vi "SW-Modbus Err Status.vi"(11 "Modbus Error Code function":i32) -> (2 "结果输出":string, 3 "Status":bool)   [LabVIEW 2015]
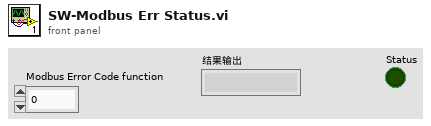
[diagram p1: front panel]
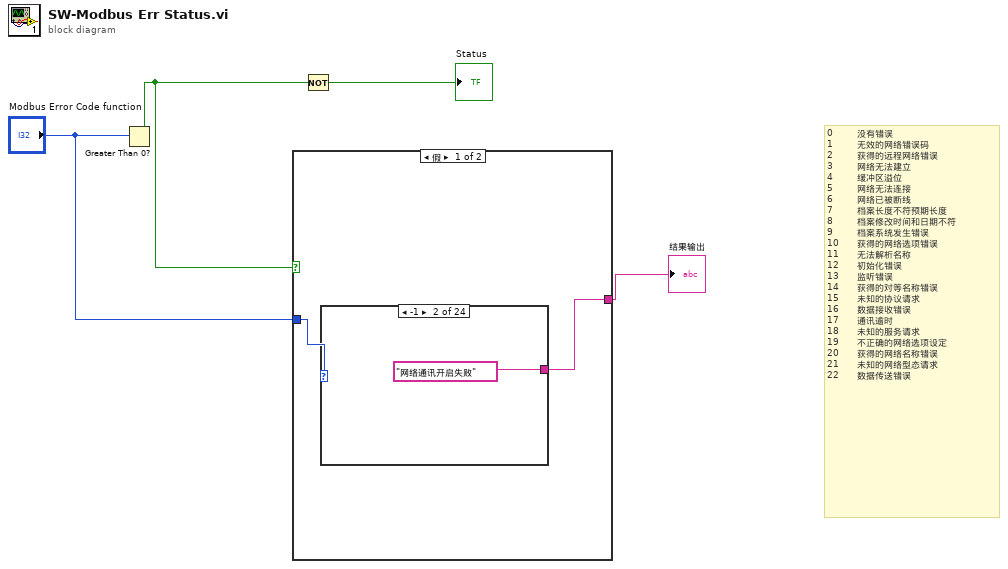
[diagram p0: block diagram]
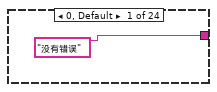
[diagram p2: hidden frame]
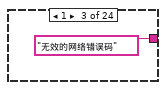
[diagram p3: hidden frame]
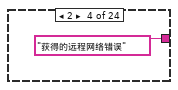
[diagram p4: hidden frame]
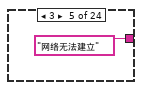
[diagram p5: hidden frame]
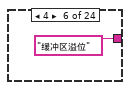
[diagram p6: hidden frame]
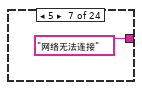
[diagram p7: hidden frame]
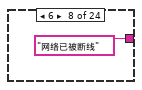
[diagram p8: hidden frame]
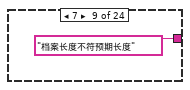
[diagram p9: hidden frame]
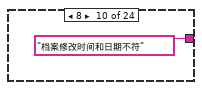
[diagram p10: hidden frame]
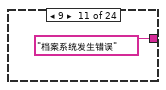
[diagram p11: hidden frame]
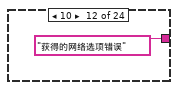
[diagram p12: hidden frame]
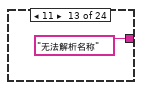
[diagram p13: hidden frame]
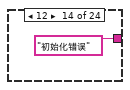
[diagram p14: hidden frame]
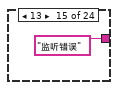
[diagram p15: hidden frame]
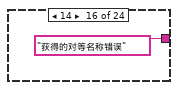
[diagram p16: hidden frame]
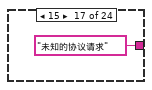
[diagram p17: hidden frame]
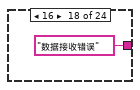
[diagram p18: hidden frame]
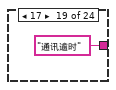
[diagram p19: hidden frame]
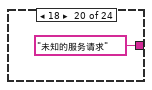
[diagram p20: hidden frame]
diagram:
  # "0        没有错误\n1        无效的网络错误码\n2        获得的远程网络错误\n3        网络无法建立\n4        缓冲区溢位\n5        网络无法连接\n6        网络已被断线\n7        档案长度不符预期长度\n8        档案修改时间和日期不符\n9        档案系统发生错误\n10      获得的网络选项错误\n11      无法解析名称\n12      初始化错误\n13      监听错误\n14      获得的对等名称错误\n15      未知的协议请求\n16      数据接收错误\n17      通讯逾时\n18      未知的服务请求\n19      不正确的网络选项设定\n20      获得的网络名称错误\n21      未知的网络型态请求\n22      数据传送错误"
  n1 = Greater Than 0?(x="Modbus Error Code function") -> (x > 0?=w2:bool)
  n2 = case shown="假" w2 {
    tunnel: "Modbus Error Code function" -> [w6 _]
    tunnel: [w5 "没有错误"] -> w3
    frame False {
      n3 = case shown="-1" w6 {
        tunnel: ["没有错误" "网络通讯开启失败" "无效的网络错误码" "获得的远程网络错误" "网络无法建立" "缓冲区溢位" "网络无法连接" "网络已被断线" "档案长度不符预期长度" "档案修改时间和日期不符" "档案系统发生错误" "获得的网络选项错误" "无法解析名称" "初始化错误" "监听错误" "获得的对等名称错误" "未知的协议请求" "数据接收错误" "通讯逾时" "未知的服务请求" "不正确的网络选项设定" "获得的网络名称错误" "未知的网络型态请求" "数据传送错误"] -> w5
        frame 0, Default {
        }
        frame -1 {
        }
        frame 1 {
        }
        frame 2 {
        }
        frame 3 {
        }
        frame 4 {
        }
        frame 5 {
        }
        frame 6 {
        }
        frame 7 {
        }
        frame 8 {
        }
        frame 9 {
        }
        frame 10 {
        }
        frame 11 {
        }
        frame 12 {
        }
        frame 13 {
        }
        frame 14 {
        }
        frame 15 {
        }
        frame 16 {
        }
        frame 17 {
        }
        frame 18 {
        }
        frame 19 {
        }
        frame 20 {
        }
        frame 21 {
        }
        frame 22 {
        }
      }
    }
    frame True {
    }
  }
  "结果输出" <- w3
  n4 = Not(x=w2) -> (.not. x?=→"Status":bool)
